vi "get_status.vi"(8 "error in (no error)":errorcluster, 11 "StageFH090410SharedVariable in":refnum<class "StageFH090410SharedVariable.lvclass">) -> (0 "error out":errorcluster, 2 "is happy?":bool, 3 "StageFH090410SharedVariable out":refnum<class "StageFH090410SharedVariable.lvclass">)   [LabVIEW 2010, in "StageFH090410SharedVariable.lvclass"]
uses:
  StageFH090410SharedVariable.lvclass
  StageFH090410SharedVariable.lvclass/StageFH090410SharedVariable.ctl
  common/classes/SpaceVector/SpaceVector/SpaceVector.lvclass
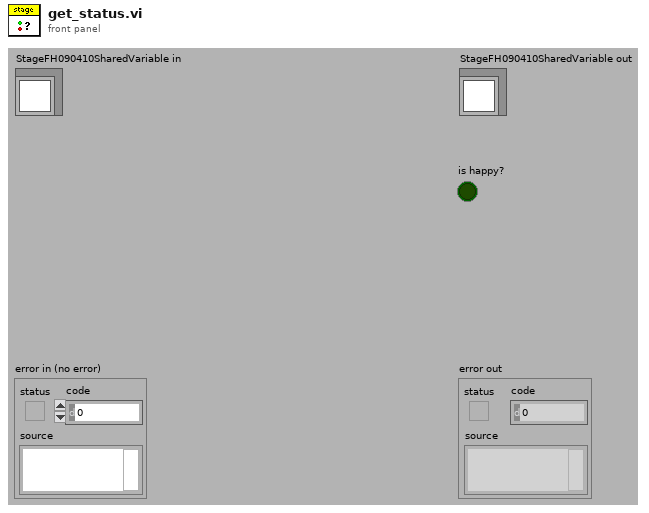
[diagram p1: front panel]
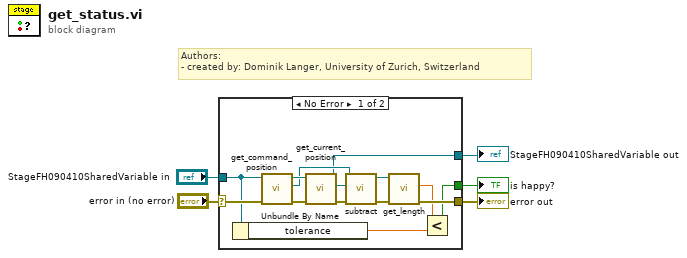
[diagram p0: block diagram]
diagram:
  # "Authors: \n- created by: Dominik Langer, University of Zurich, Switzerland"
  n1 = case shown="No Error" "error in (no error)" {
    selector: "error in (no error)" -> [w18 w20]
    tunnel: "StageFH090410SharedVariable in" -> [w6 w19]
    tunnel: [w8 w19] -> w3
    tunnel: [w11 w20] -> w2
    tunnel: [w9 _] -> w1
    frame No Error {
      n2 = Unbundle By Name(w6) -> ("tolerance"=w7:dbl[unit])
      n3 = call-dynamic "get_command_position.vi"("error in (no error)"=w18, "DL090409StageScaffold.lvclass in"=w6) -> ("error out"=w14:errorcluster, "SpaceVector.lvclass"=w16:refnum<class "SpaceVector.lvclass">, "DL090409StageScaffold.lvclass out"=w17:refnum<class "StageFH090410SharedVariable.lvclass">)  [unwired: 7 in]
      n4 = call-dynamic "get_current_position.vi"("DL090409StageScaffold.lvclass in"=w17) -> ("current position"=w15:refnum<class "SpaceVector.lvclass">, "DL090409StageScaffold.lvclass out"=w8:refnum<class "StageFH090410SharedVariable.lvclass">)  [unwired: 8 in, 1 out]
      n5 = call "subtract.vi"("error in (no error)"=w14, "subtrahend"=w15, "SpaceVector in"=w16) -> ("error out"=w12:errorcluster, "SpaceVector out"=w13:refnum<class "SpaceVector.lvclass">)  [unwired: 7 in]
      n6 = call "get_length.vi"("error in (no error)"=w12, "SpaceVector in"=w13) -> ("error out"=w11:errorcluster, "length"=w10:dbl[unit])  [unwired: 7 in, 1 out]
      n7 = Less?(x=w10, y=w7) -> (x < y?=w9:bool)
    }
    frame Error {
    }
  }
  "error out" <- w2
  "StageFH090410SharedVariable out" <- w3
  "is happy?" <- w1
